vi "TrajectoryGenerate_splinePointsFromSplines.vi"(11 "inputSPLINE":T1[](array[typedef])) -> (0 "error out":errorcluster, 3 "ArrayPoseWithCurvature":T3[](array[typedef]) {"POSE"."ROTATION"."SIN" format="%13.4f"; "POSE"."ROTATION"."COS" format="%13.4f"; "POSE"."ROTATION"."VALUE" format="%13.4f"; "POSE"."TRANSLATION"."Y" format="%14.3f"; "POSE"."TRANSLATION"."X" format="%14.3f"})   [LabVIEW 2019, in "Trajectory_Library.lvlib"]
doc: "Generate spline points from a vector of splines by parameterizing the splines.\n \nParameters:\n - inputSpline - Array of splines to parameterize.\n\nReturns:\n - ArrayPoseWithCurvature - The spline points for use in time parameterization of a trajectory.\n - Error Out - Returned error cluster"
uses:
  Trajectory_Library.lvlib
  TypeDef/TRANSLATION2D.ctl
  TypeDef/ROTATION2D.ctl
  TypeDef/POSE2D.ctl
  TypeDef/POSEwCURVATURE.ctl
  <vilib>/Analysis/Matrix/Datatypes/RealMatrix.ctl
  <vilib>/Analysis/Matrix/NI_Matrix.lvlib
  TypeDef/SPLINE.ctl
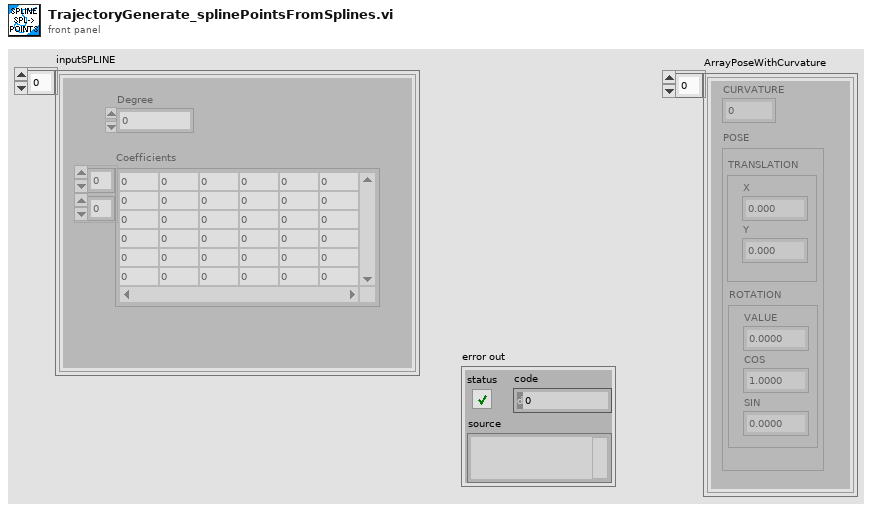
[diagram p1: front panel]
types:
  T1 = typedef "Trajectory_Library.lvlib/SPLINE.ctl" = cluster{"Degree":i32, "Coefficients":T2}
  T2 = typedef "NI_Matrix.lvlib/RealMatrix.ctl" = dbl[][]
  T3 = typedef "Trajectory_Library.lvlib/POSEwCURVATURE.ctl" = cluster{"CURVATURE":dbl, "POSE":T4}
  T4 = typedef "Trajectory_Library.lvlib/POSE2D.ctl" = cluster{"TRANSLATION":T5, "ROTATION":T6}
  T5 = typedef "Trajectory_Library.lvlib/TRANSLATION2D.ctl" = cluster{"X":dbl, "Y":dbl}
  T6 = typedef "Trajectory_Library.lvlib/ROTATION2D.ctl" = cluster{"VALUE":dbl, "COS":dbl, "SIN":dbl}
  T7 = typedef "WPILib_Math.lvlib/POSEwCURVATURE.ctl" = cluster{"CURVATURE":dbl, "POSE":T8}
  T8 = typedef "WPILib_Math.lvlib/POSE2D.ctl" = cluster{"TRANSLATION":T9, "ROTATION":T10}
  T9 = typedef "WPILib_Math.lvlib/TRANSLATION2D.ctl" = cluster{"X":dbl, "Y":dbl}
  T10 = typedef "WPILib_Math.lvlib/ROTATION2D.ctl" = cluster{"VALUE":dbl, "COS":dbl, "SIN":dbl}
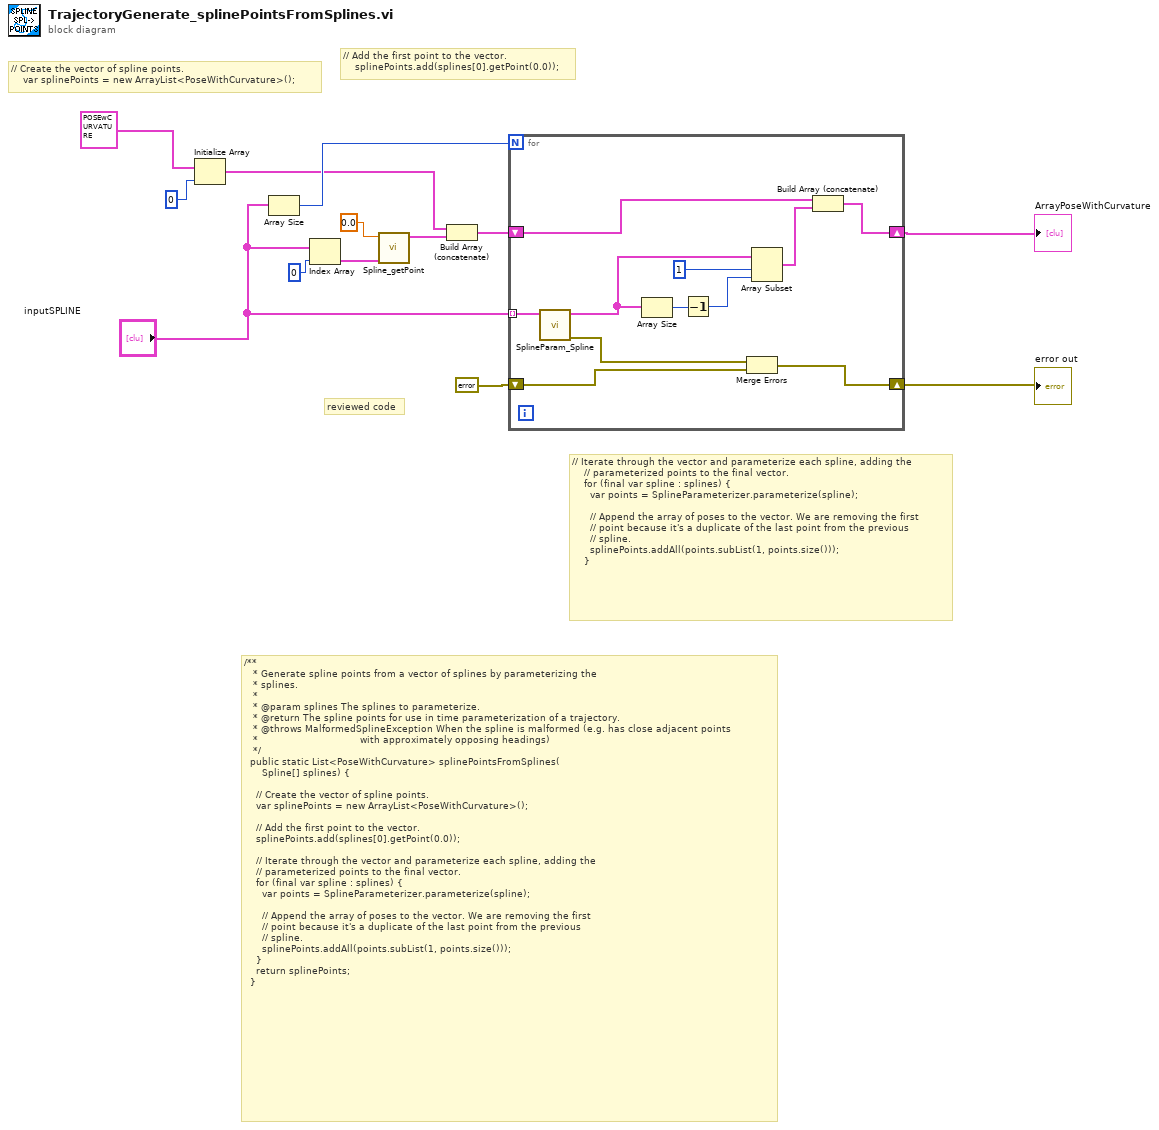
[diagram p0: block diagram]
diagram:
  # "reviewed code"
  # "// Iterate through the vector and parameterize each spline, adding the\n    // parameterized points to the final vector.\n    for (final var spline : splines) {\n      var points = SplineParameterizer.parameterize(spline);\n\n      // Append the array of poses to the vector. We are removing the first\n      // point because it's a duplicate of the last point from the previous\n      // spline.\n      splinePoints.addAll(points.subList(1, points.size()));\n    }"
  # "// Add the first point to the vector.\n    splinePoints.add(splines[0].getPoint(0.0));"
  # "// Create the vector of spline points.\n    var splinePoints = new ArrayList<PoseWithCurvature>();"
  # "/**\n   * Generate spline points from a vector of splines by parameterizing the\n   * splines.\n   *\n   * @param splines The splines to parameterize.\n   * @return The spline points for use in time parameterization of a trajectory.\n   * @throws MalformedSplineException When the spline is malformed (e.g. has close adjacent points\n   *                                  with approximately opposing headings)\n   */\n  public static List<PoseWithCurvature> splinePointsFromSplines(\n      Spline[] splines) {\n\n    // Create the vector of spline points.\n    var splinePoints = new ArrayList<PoseWithCurvature>();\n\n    // Add the first point to the vector.\n    splinePoints.add(splines[0].getPoint(0.0));\n\n    // Iterate through the vector and parameterize each spline, adding the\n    // parameterized points to the final vector.\n    for (final var spline : splines) {\n      var points = SplineParameterizer.parameterize(spline);\n\n      // Append the array of poses to the vector. We are removing the first\n      // point because it's a duplicate of the last point from the previous\n      // spline.\n      splinePoints.addAll(points.subList(1, points.size()));\n    }\n    return splinePoints;\n  }"
  n1 = Initialize Array(T3 {"CURVATURE"=0.0, "POSE"={"TRANSLATION"={"X"=0.0, "Y"=0.0}, "ROTATION"={"VALUE"=0.0, "COS"=1.0, "SIN"=0.0}}} ("POSEwCURVATURE"), 0 ("dimension size")) -> (w2:T3[])
  n2 = Array Size(array="inputSPLINE") -> (size(s)=w10:i32)
  n3 = Index Array(array="inputSPLINE", index=0) -> (element=w11:T1)
  n4 = call "Spline_getPoint.vi"("inputSPLINE"=w11, "Time"=0.0) -> ("POSEwCURVATURE"=w1:T7)  [unwired: 9 in]
  n5 = Build Array (concatenate)(w2, w1) -> (w3:T7[])
  n6 = for {
    N: w10 -> [_]
    shift-right: [w19] -> w6
    shift-left: w3 -> [w20]
    tunnel: "inputSPLINE" -> [w24] mode=indexing
    shift-right: [w23] -> w4
    shift-left: errorcluster {"status"=FALSE, "code"=0, "source"=""} ("error out") -> [w22]
    n7 = call "SplineParam_Spline.vi"("inputSPLINE"=w24) -> ("error out"=w21:errorcluster, "outputPOSEwCURVATURE"=w18:T7[])  [unwired: 9 in]
    n8 = Array Size(array=w18) -> (size(s)=w16:i32)
    n9 = Decrement(x=w16) -> (x-1=w15:i32)
    n10 = Merge Errors(w21, w22) -> (w23:errorcluster)
    n11 = Array Subset(array=w18, index=1, length=w15) -> (w14:T7[])
    n12 = Build Array (concatenate)(w20, w14) -> (w19:T7[])
  }
  "error out" <- w4
  "ArrayPoseWithCurvature" <- w6
